vi "SLSC Refresh Tree Control.vi"(4 "SLSCChannelPath":string="SLSCChannelPath", 5 "Update Only?":bool, 6 "enums":T2[](array[typedef]), 7 "TreeControl in":refnum<vi>, 8 "error in (no error)":errorcluster, 9 "SLSC Output Tree":T3(array[cluster]), 11 "Item Ref in":T1 format="%.0x") -> (0 "error out":errorcluster, 3 "Item Ref in 2":T1 format="%.0x")   [LabVIEW 2017, in "SLSC EDS System Explorer.lvlib"]
uses:
  SLSC EDS System Explorer.lvlib
  <vilib>/NI Veristand/Custom Device API/Custom Device Item Ref.ctl
  SLSC EDS API/JSON parsing/enum.ctl
  SLSC UI API/SLSC Tree Control.lvlib
  SLSC CD API/SLSC CD System Explorer/SLSC CD System Explorer.lvlib
  <vilib>/NI VeriStand/Custom Device API/Custom Device API.lvlib
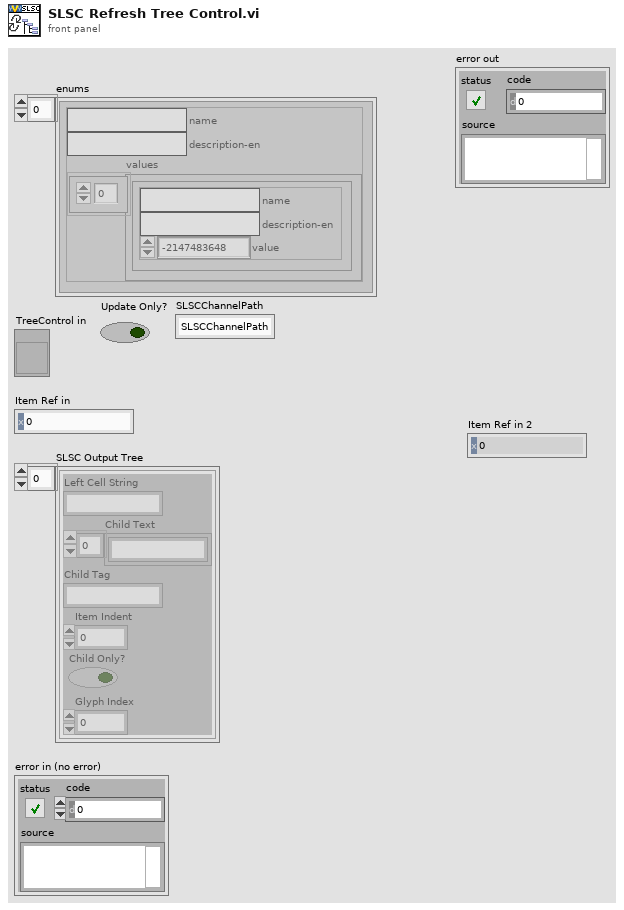
[diagram p1: front panel]
types:
  T1 = typedef "Custom Device API.lvlib/Custom Device Item Ref.ctl" = u64
  T2 = typedef "enum.ctl" = cluster{"name":string, "description-en":string, "values":cluster{"name":string, "description-en":string, "value":i32}[]}
  T3 = cluster{"Left Cell String":string, "Child Text":string[], "Child Tag":string, "Item Indent":i32, "Child Only?":bool, "Glyph Index":i32}[]
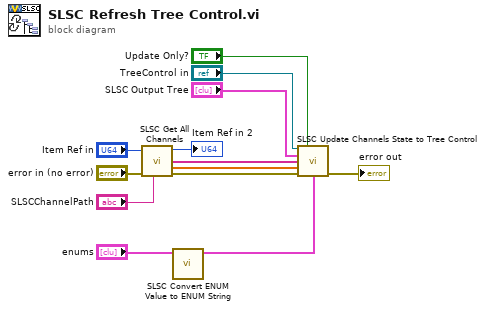
[diagram p0: block diagram]
diagram:
  n1 = call "SLSC Get All Channels.vi"("SLSCChannelPath"="SLSCChannelPath", "error in (no error)"="error in (no error)", "Item Ref in"="Item Ref in") -> ("error out"=w2:errorcluster, "Channel Values"=w3:dbl[], "TreeItem Channels"=w10:string[], "Item Ref out"=→"Item Ref in 2":T1)  [unwired: 5 in]
  n2 = call "SLSC Convert ENUM Value to ENUM String.vi"("Enums"="enums") -> ("String Enums"=w4:cluster{"name":string, "string enums":string}[])  [unwired: 9 in, 1 out]
  n3 = call "SLSC Update Channels State to Tree Control.vi"("Property tree"="TreeControl in", "Update Only?"="Update Only?", "SLSC Output Tree"="SLSC Output Tree", "Channels to \"enable\""=w10, "Channel Values"=w3, "error in (no error)"=w2, "Enum Strings"=w4) -> ("error out"=→"error out":errorcluster)  [unwired: 8 in]
